vi "SetList Columns to Devices.vi"(8 "error in (no error)":errorcluster, 9 "Col array in":refnum<class "Column.lvclass">[](array[class]), 10 "DevNums In":i32[](array[numeric]), 11 "Devices queue":refnum<queue>) -> (0 "error out":errorcluster, 3 "Devices queue out":refnum<queue>)   [LabVIEW 2013]
doc: "Loop over devices and set corresponding columns from Table's column array. (Appearance only, not SWI data!)\nThis VI is read-only w.r.t column data."
uses:
  ColumnVIs/Column/Column.lvclass
  Device/Device.lvclass
panel:
  # "Want to update SetList Appearance changes to devices!"
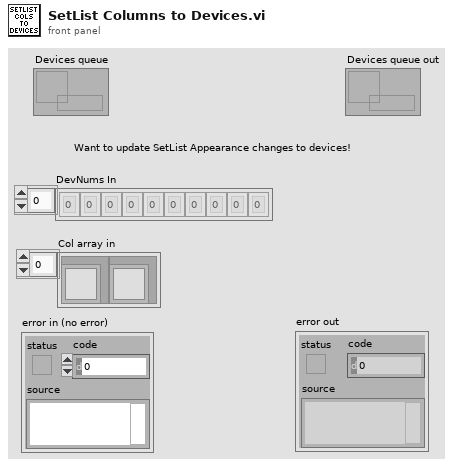
[diagram p1: front panel]
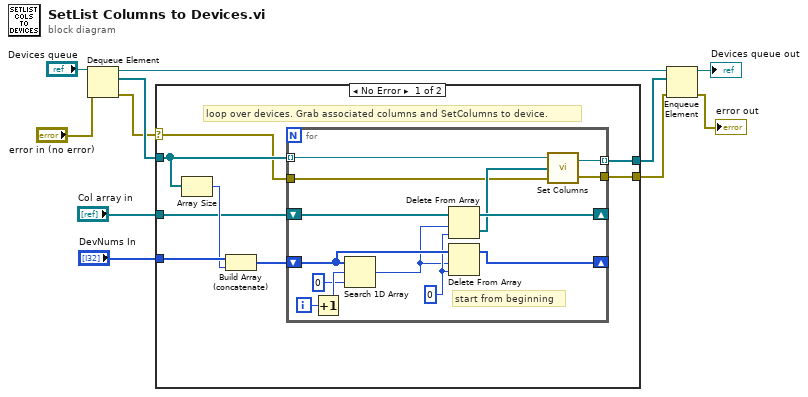
[diagram p0: block diagram]
diagram:
  n1 = Dequeue Element(queue="Devices queue", error in (no error)="error in (no error)") -> (queue out=w7:refnum<queue>, element=w8:refnum<class "Device.lvclass">[], error out=w2:errorcluster)  [unwired: 1 in, 1 out]
  n2 = case shown="No Error" w2 {
    selector: w2 -> [w12 w35]
    tunnel: [w19 w34] -> w6
    tunnel: w8 -> [w18 w34]
    tunnel: "DevNums In" -> [w17 _]
    tunnel: "Col array in" -> [w14 _]
    tunnel: [w13 w35] -> w4
    frame No Error {
      # "loop over devices. Grab associated columns and SetColumns to device."
      n3 = Array Size(array=w18) -> (size(s)=w15:i32)
      n4 = Build Array (concatenate)(w17, w15) -> (w16:i32[])
      n5 = for {
        tunnel: w18 -> [w33] mode=indexing
        tunnel: [w32] -> w19 mode=indexing
        shift-right: [w28] -> _
        shift-left: w14 -> [w29]
        shift-right: [w25] -> _
        shift-left: w16 -> [w26]
        tunnel: [w21] -> w13
        tunnel: w12 -> [w20]
        i -> [w31]
        w23 = 0 ("start index (0)")
        # "start from beginning"
        n6 = Increment(x=w31) -> (x+1=w30:i32)
        n7 = Search 1D Array(1D array=w26, element=w30, start index (0)=0) -> (index of element=w22:i32)
        n8 = Delete From Array(array=w29, length=w22, index=w23) -> (deleted portion=w27:refnum<class "Column.lvclass">[], array with subset deleted=w28:refnum<class "Column.lvclass">[])
        n9 = Delete From Array(array=w26, length=w22, index=w23) -> (array with subset deleted=w25:i32[])  [unwired: 1 out]
        n10 = call-dynamic "Set Columns.vi"("error in (no error)"=w20, "Columns"=w27, "Device in"=w33) -> ("error out"=w21:errorcluster, "Device out"=w32:refnum<class "Device.lvclass">)  [unwired: 1 in]
      }
    }
    frame Error {
    }
  }
  n11 = Enqueue Element(queue=w7, element=w6, error in (no error)=w4) -> (queue out=→"Devices queue out":refnum<queue>, error out=→"error out":errorcluster)  [unwired: 1 in, 1 out]
